vi "stave HDI measure shih v0.vi"() -> ()   [LabVIEW 2016]
uses:
  <vilib>/Utility/file.llb/Read Delimited Spreadsheet (DBL).vi
  <vilib>/Utility/file.llb/Write Delimited Spreadsheet (DBL).vi
  Classes/Controllers/Motion/Copy of Motion Folder/Motion.lvclass
  Classes/Controllers/Camera/Copy of Controller Folder/Controller.lvclass
panel:
  out "txt check":dbl[][](array[numeric])
  in  "north first switch":bool
  out "position from OGP all":dbl[][][](array[numeric]) format="%#_8g"
  out "HDI-stave deviation all":dbl[][][](array[numeric]) format="%#_8g"
  out "HDI - stave deviation on time":dbl[][](array[numeric]) format="%#_8g"
  out "position from OGP on time":dbl[][](array[numeric]) format="%#_8g"
  in  "default south HDI upper left":dbl[](array[numeric])=[448.322, 976.582, 74.9872, 0.000191129]
  in  "test":bool
  in  "how much HDI":i32=2
  out "bottom right":dbl[][](array[numeric]) format="%#_8g"
  out "bottom left":dbl[][](array[numeric]) format="%#_8g"
  out "top left":dbl[][](array[numeric]) format="%#_8g"
  out "HDI center position":dbl[][](array[numeric]) format="%#_8g"
  in  "default north HDI upper left":dbl[](array[numeric])=[448.322, 976.582, 74.9872, 0.000191129]
  in  "Default HDI size":dbl[](array[numeric])=[24.2437, 231.446, -0.099339, 0.000191129]
  out "measure times":dbl
  in  "Parking position":dbl[](array[numeric])=[625.0, 625.0, 0.0, 0.01]
  in  "measure HDI position":bool
  in  "calculate":bool
  in  "go to park":bool
  in  "stop":bool
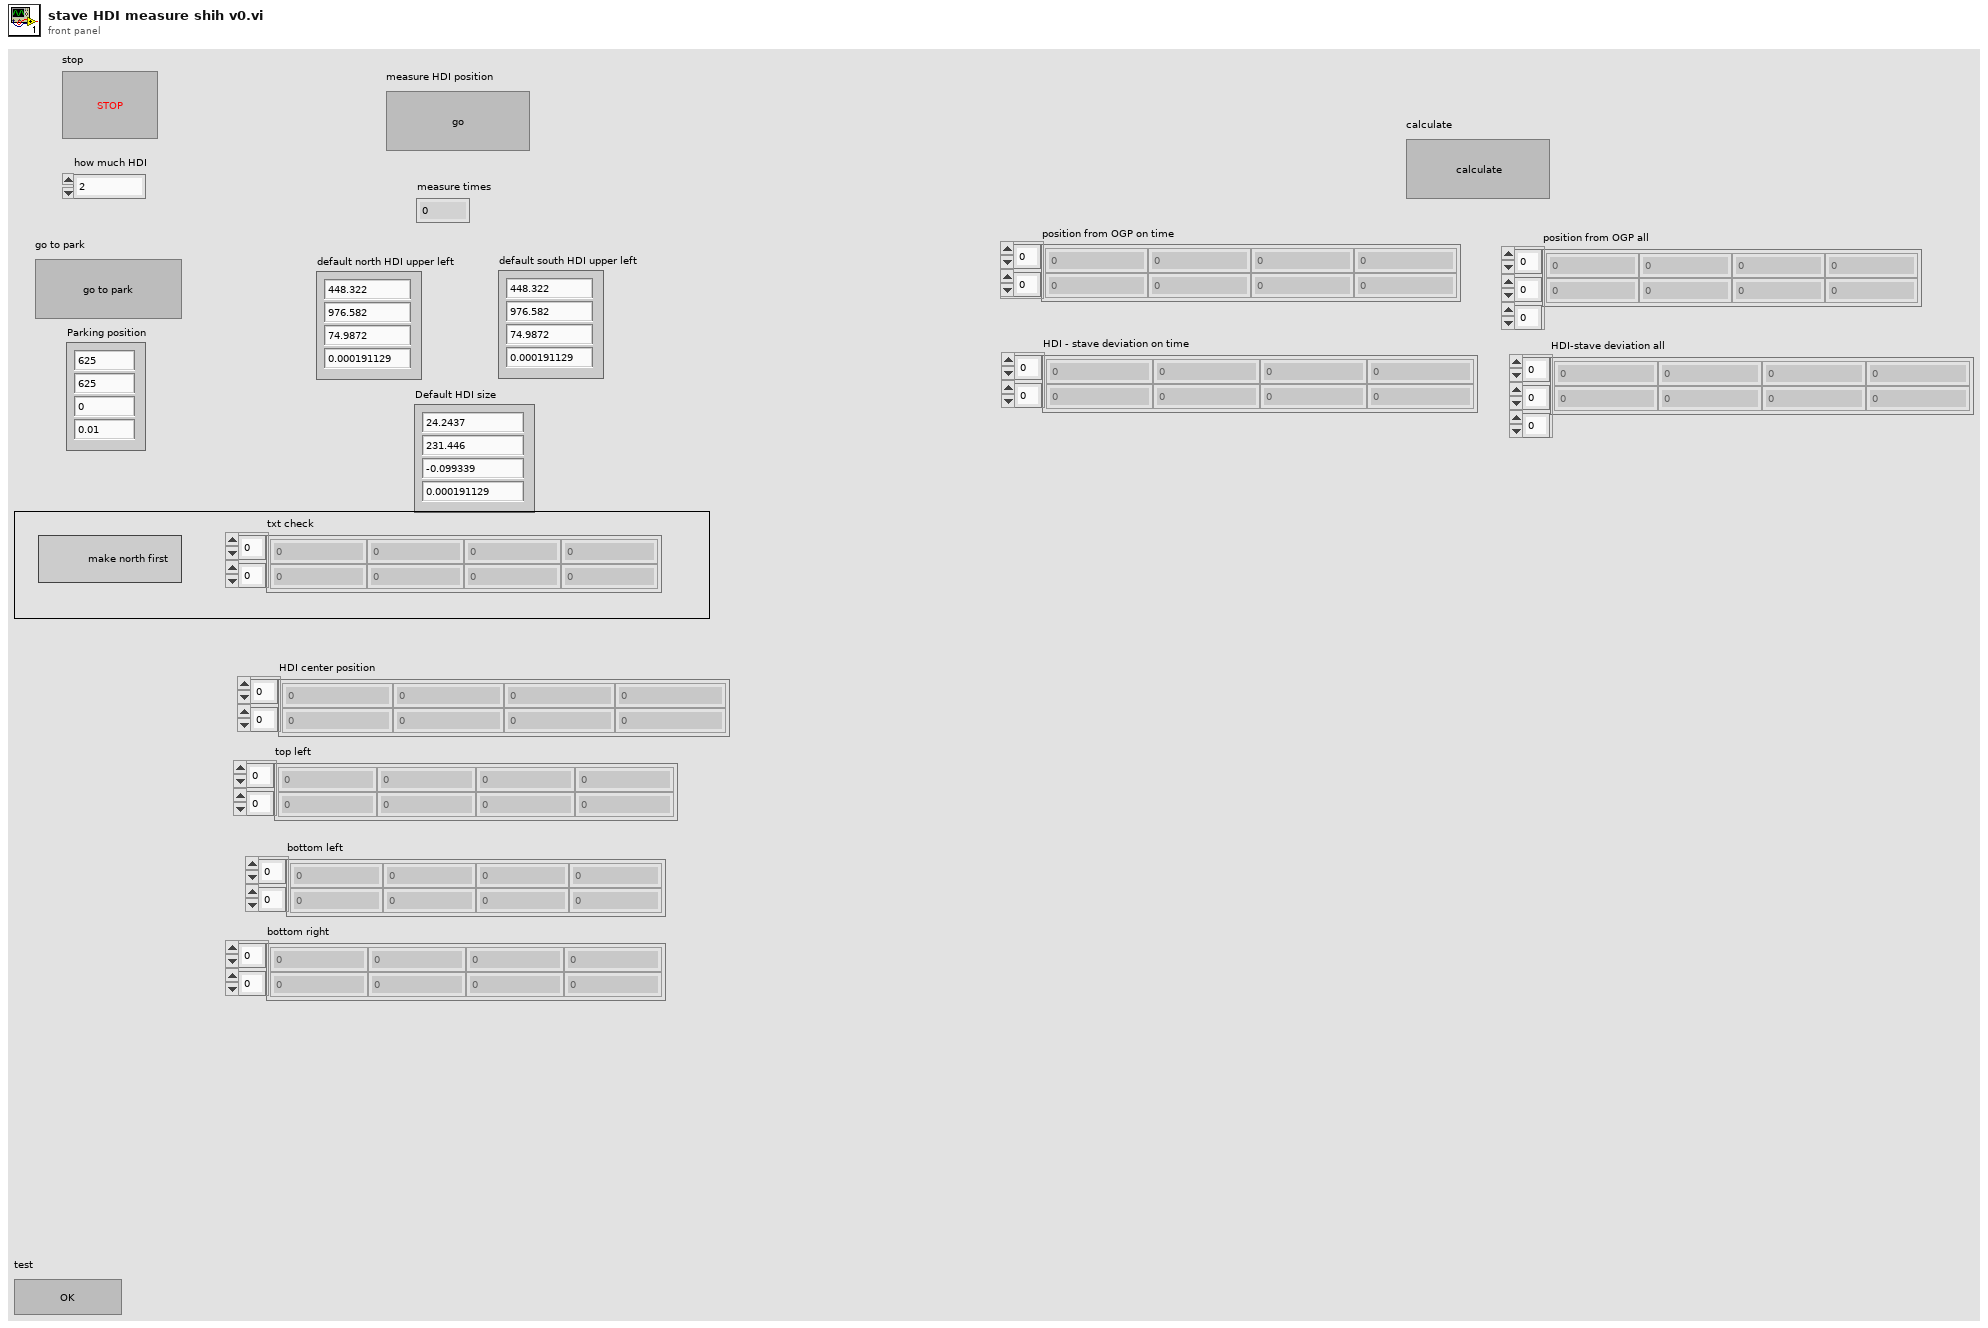
[diagram p1: front panel]
types:
  T1 = typedef "Controller.lvclass/Controllers.ctl" = cluster{"Copy of Motion.lvclass":refnum<class "Motion.lvclass">, "Copy of I-O.lvclass":refnum<class "I-O.lvclass">, "Copy of Dispenser.lvclass":refnum<class "Dispenser.lvclass">}
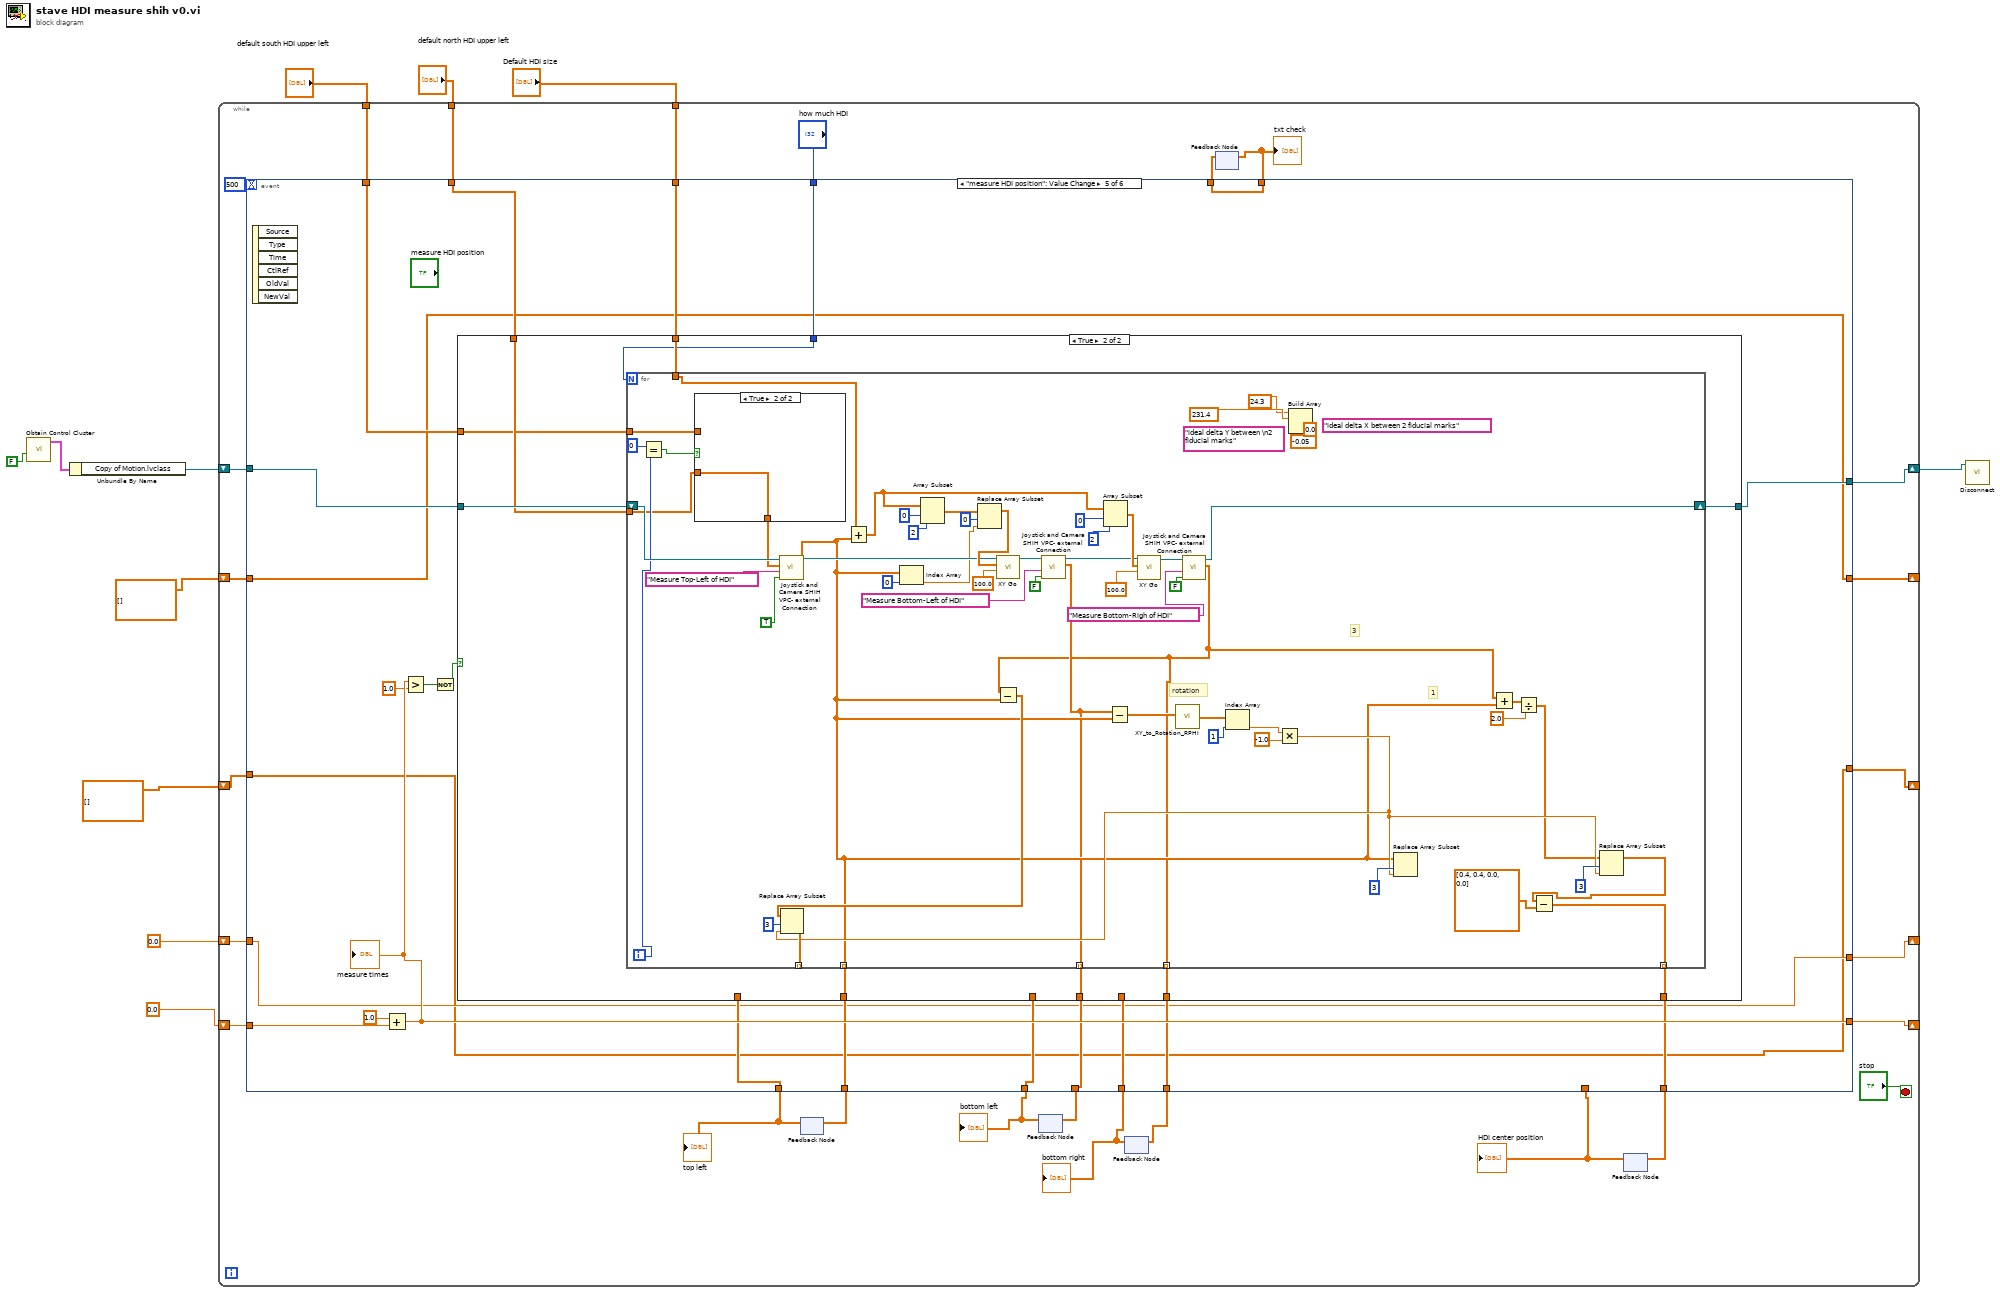
[diagram p0: block diagram]
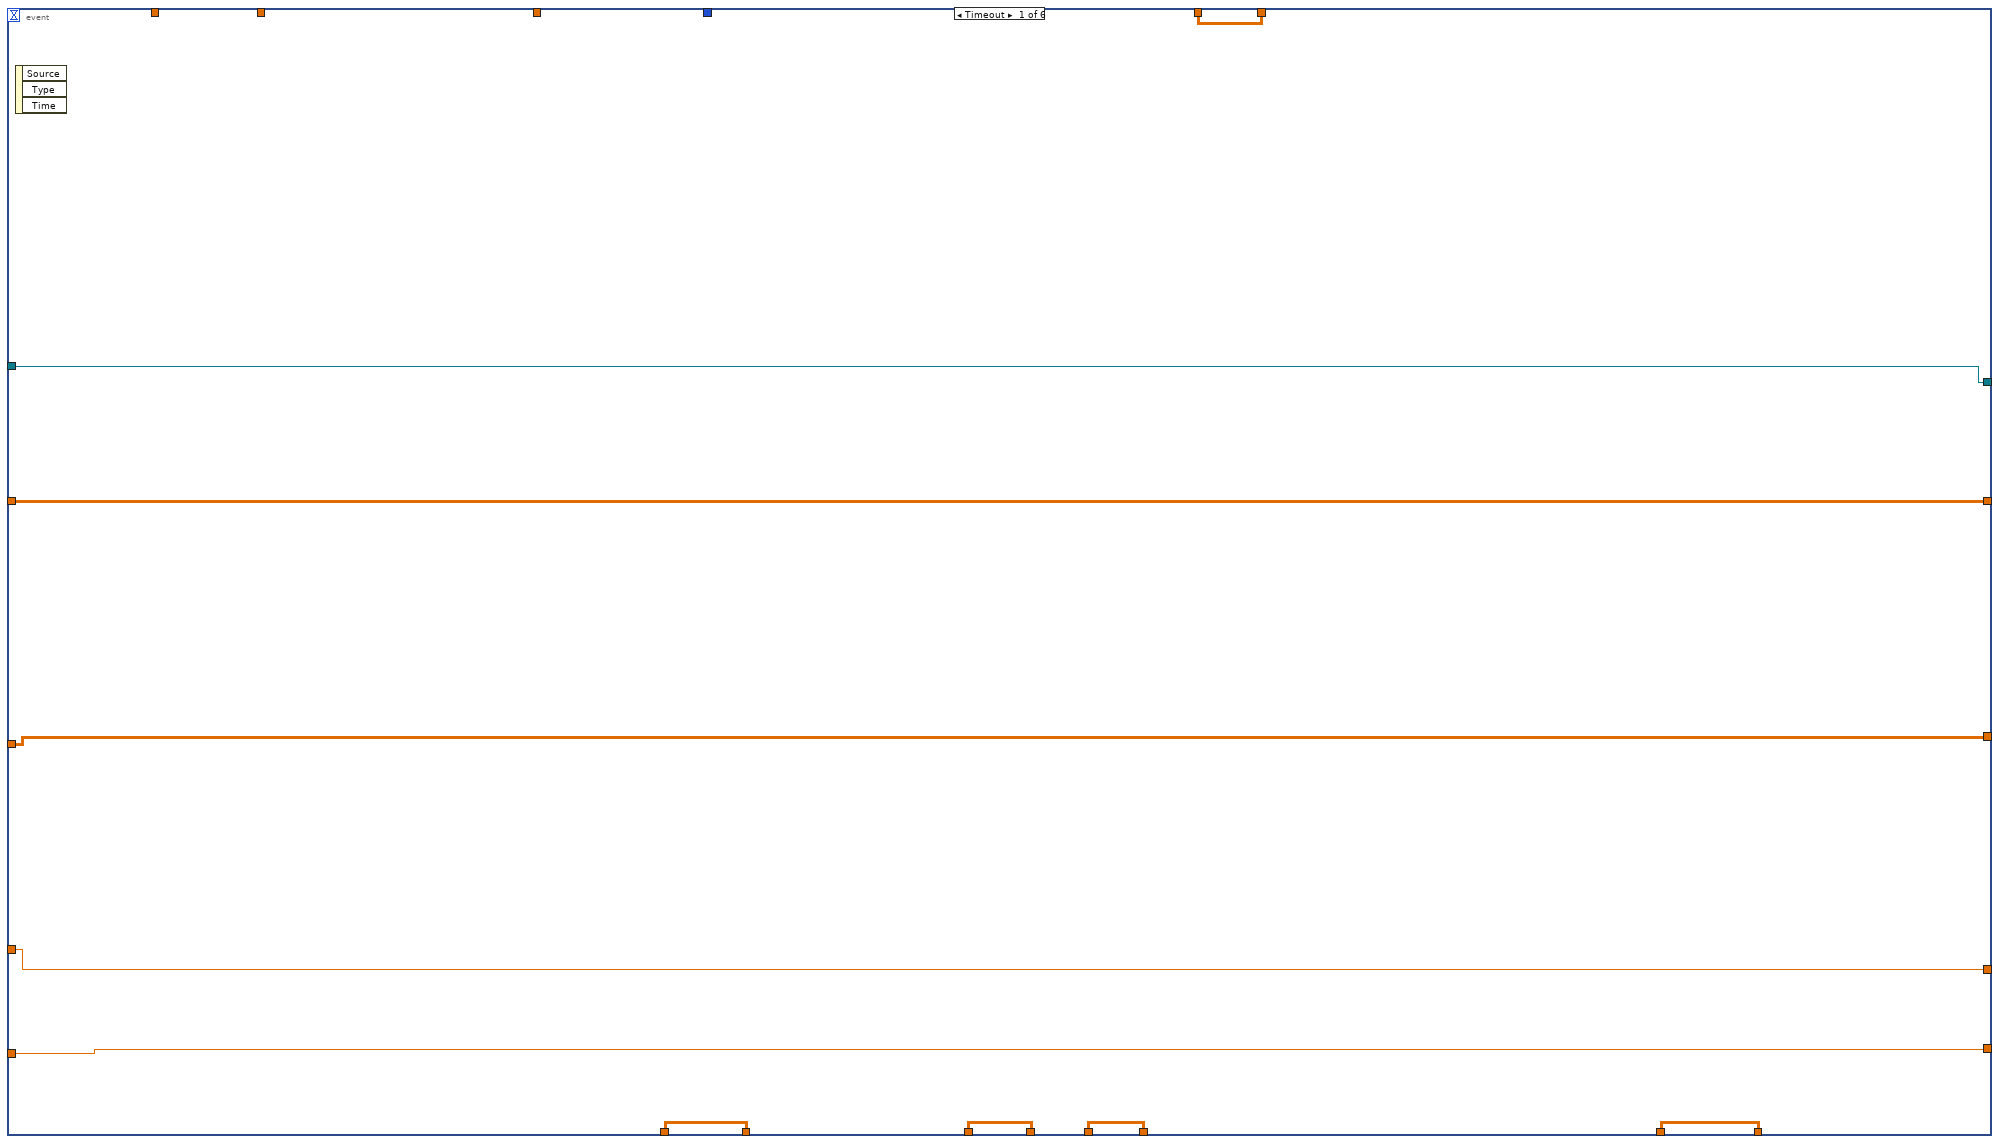
[diagram p2: hidden frame]
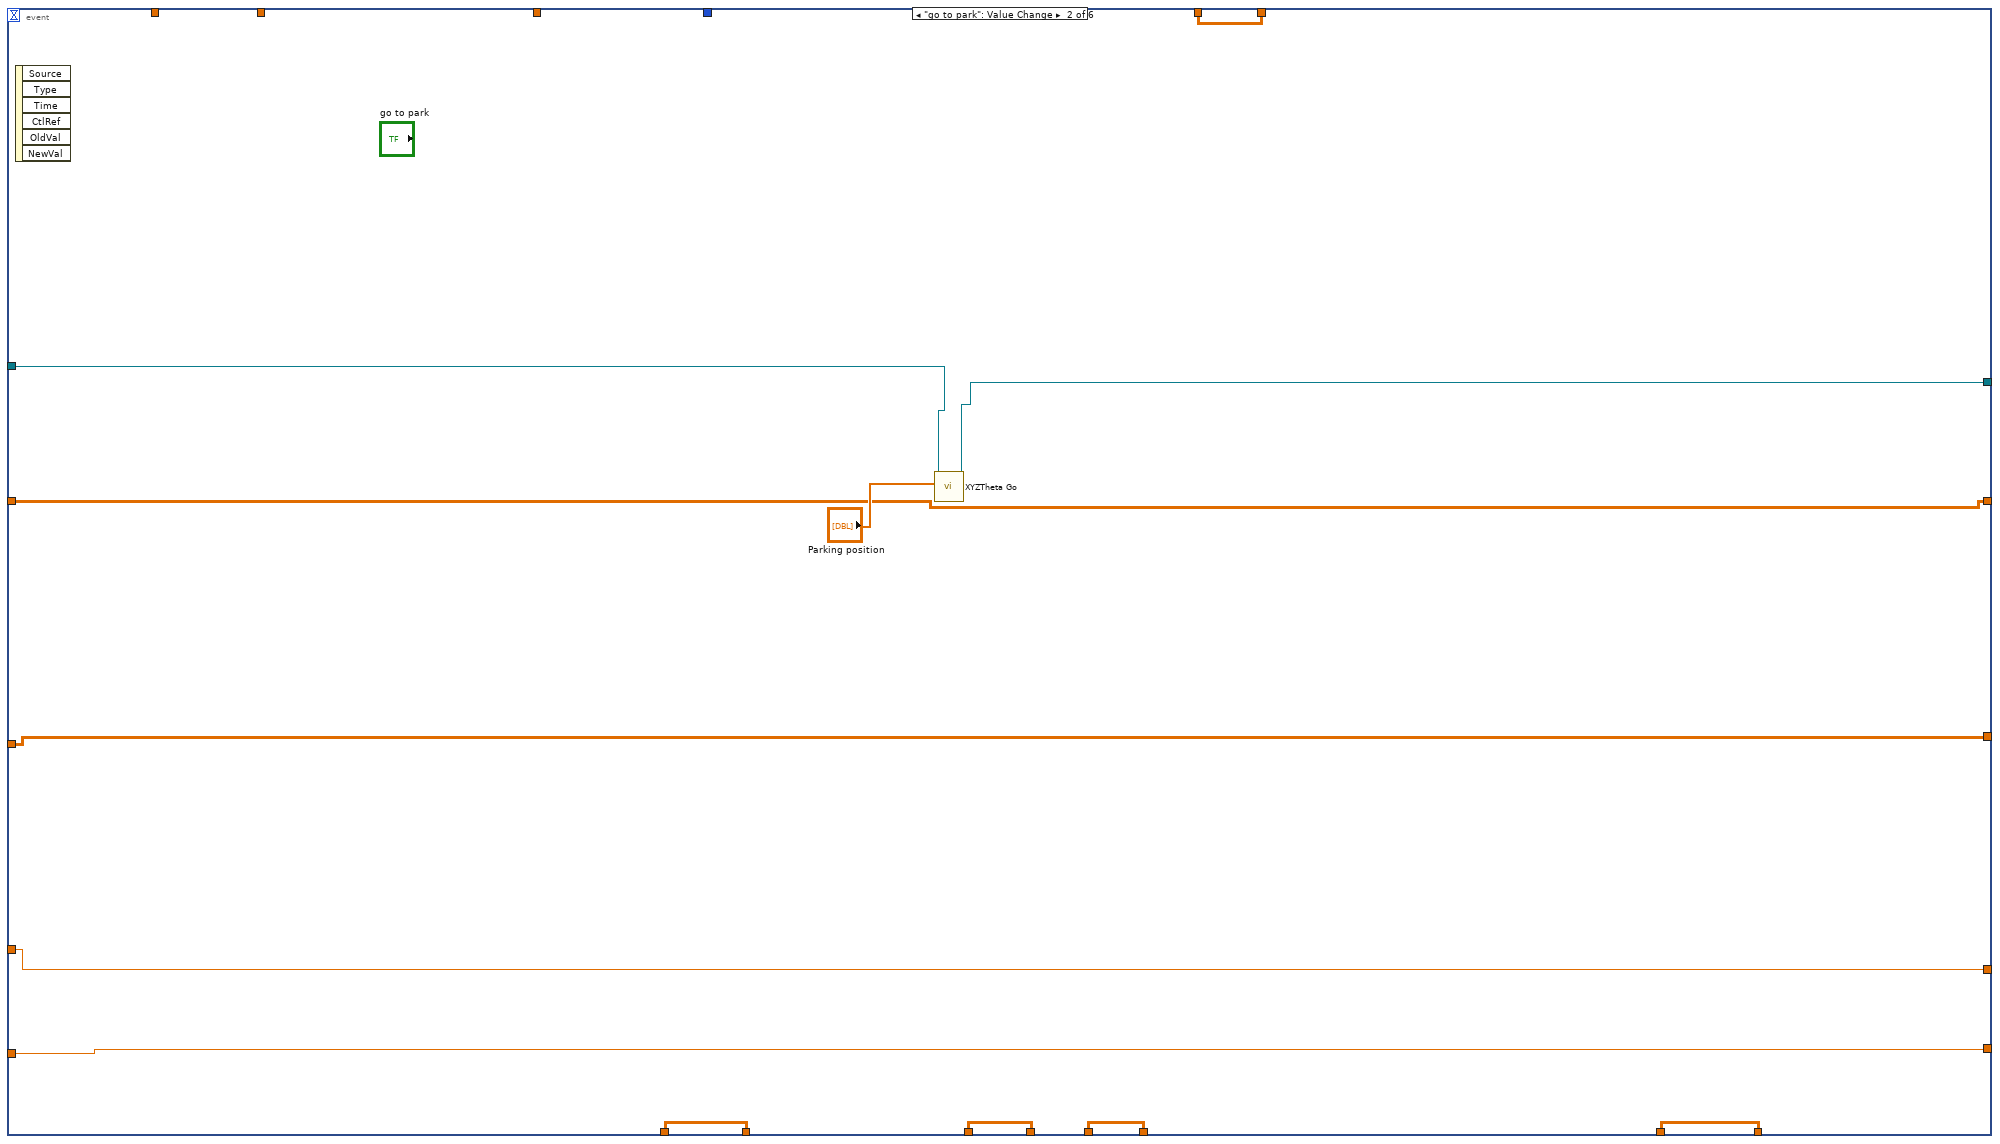
[diagram p3: hidden frame]
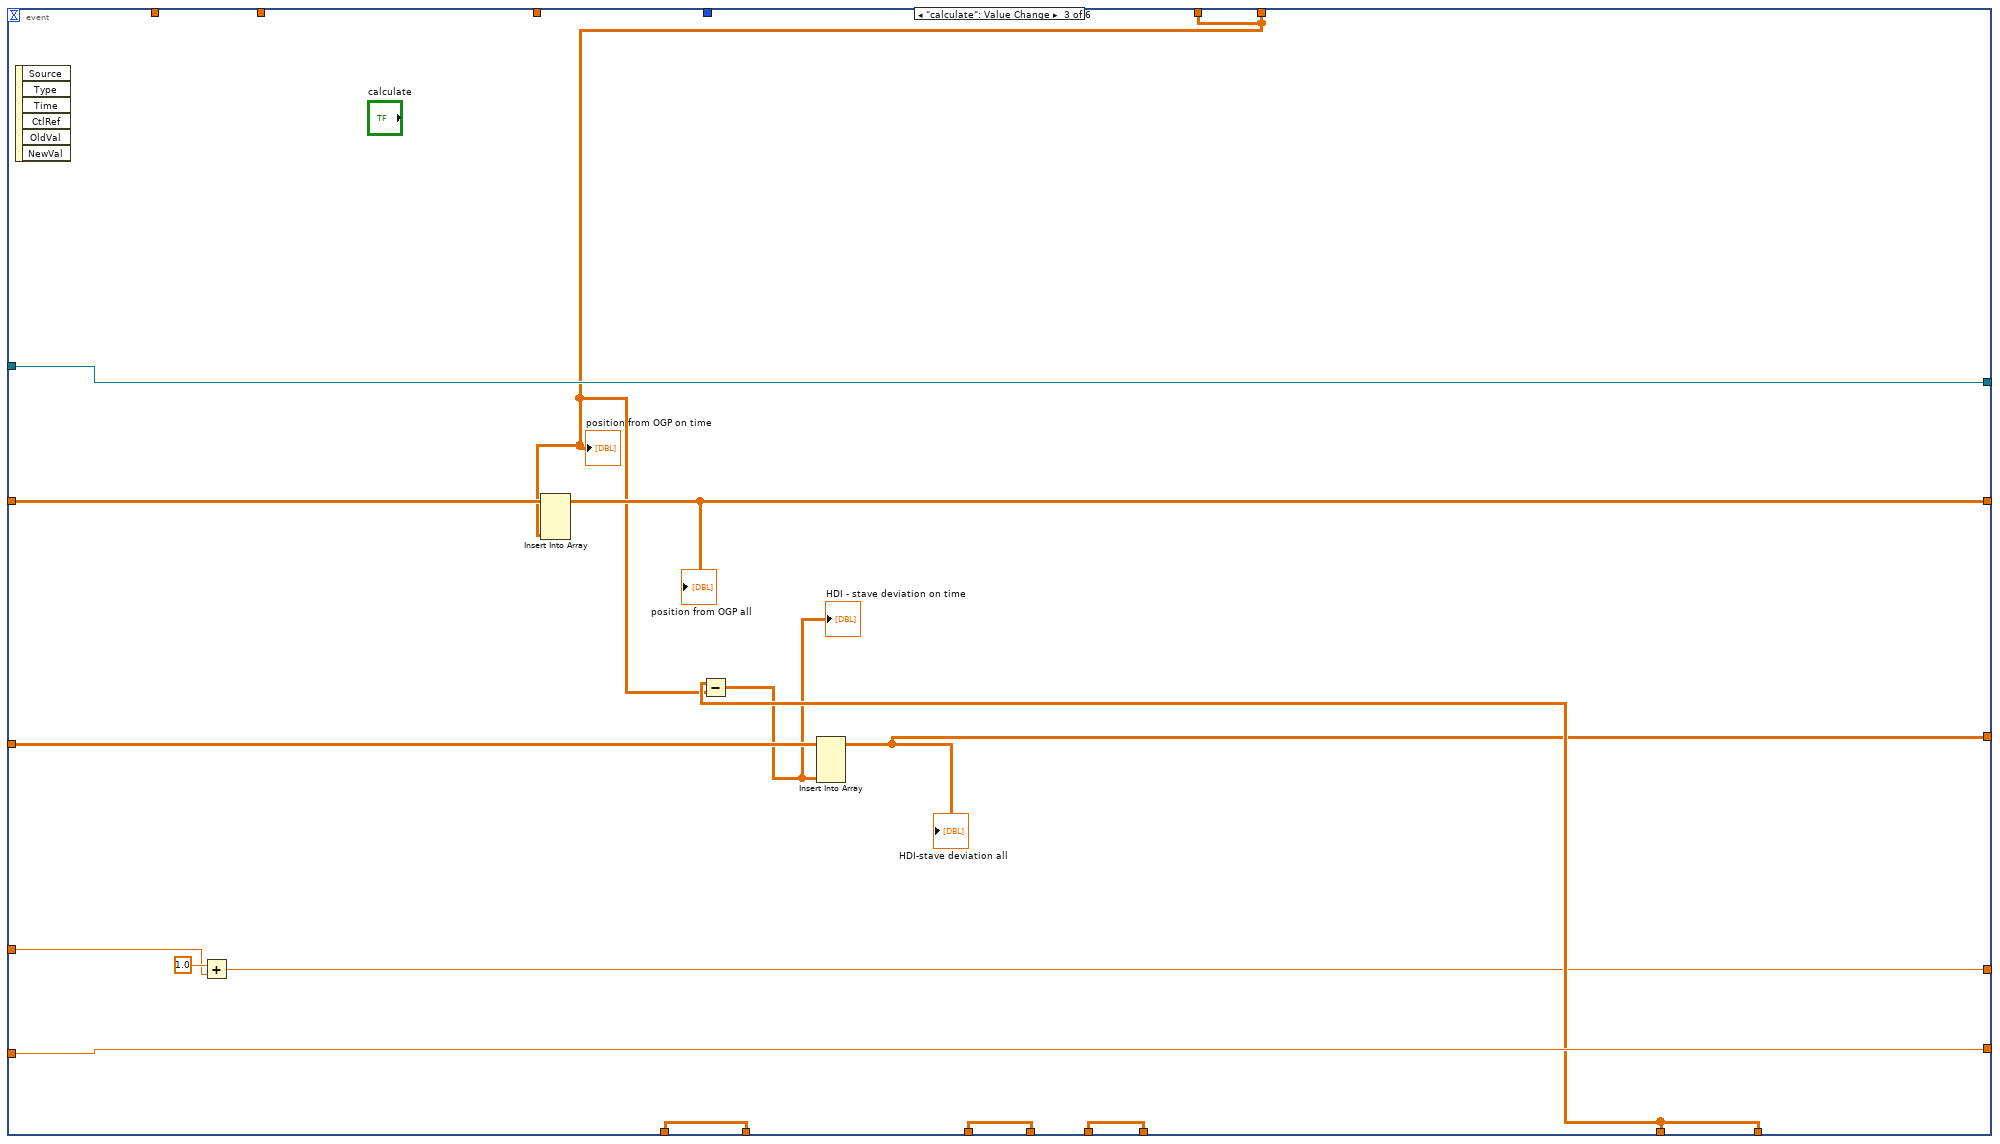
[diagram p4: hidden frame]
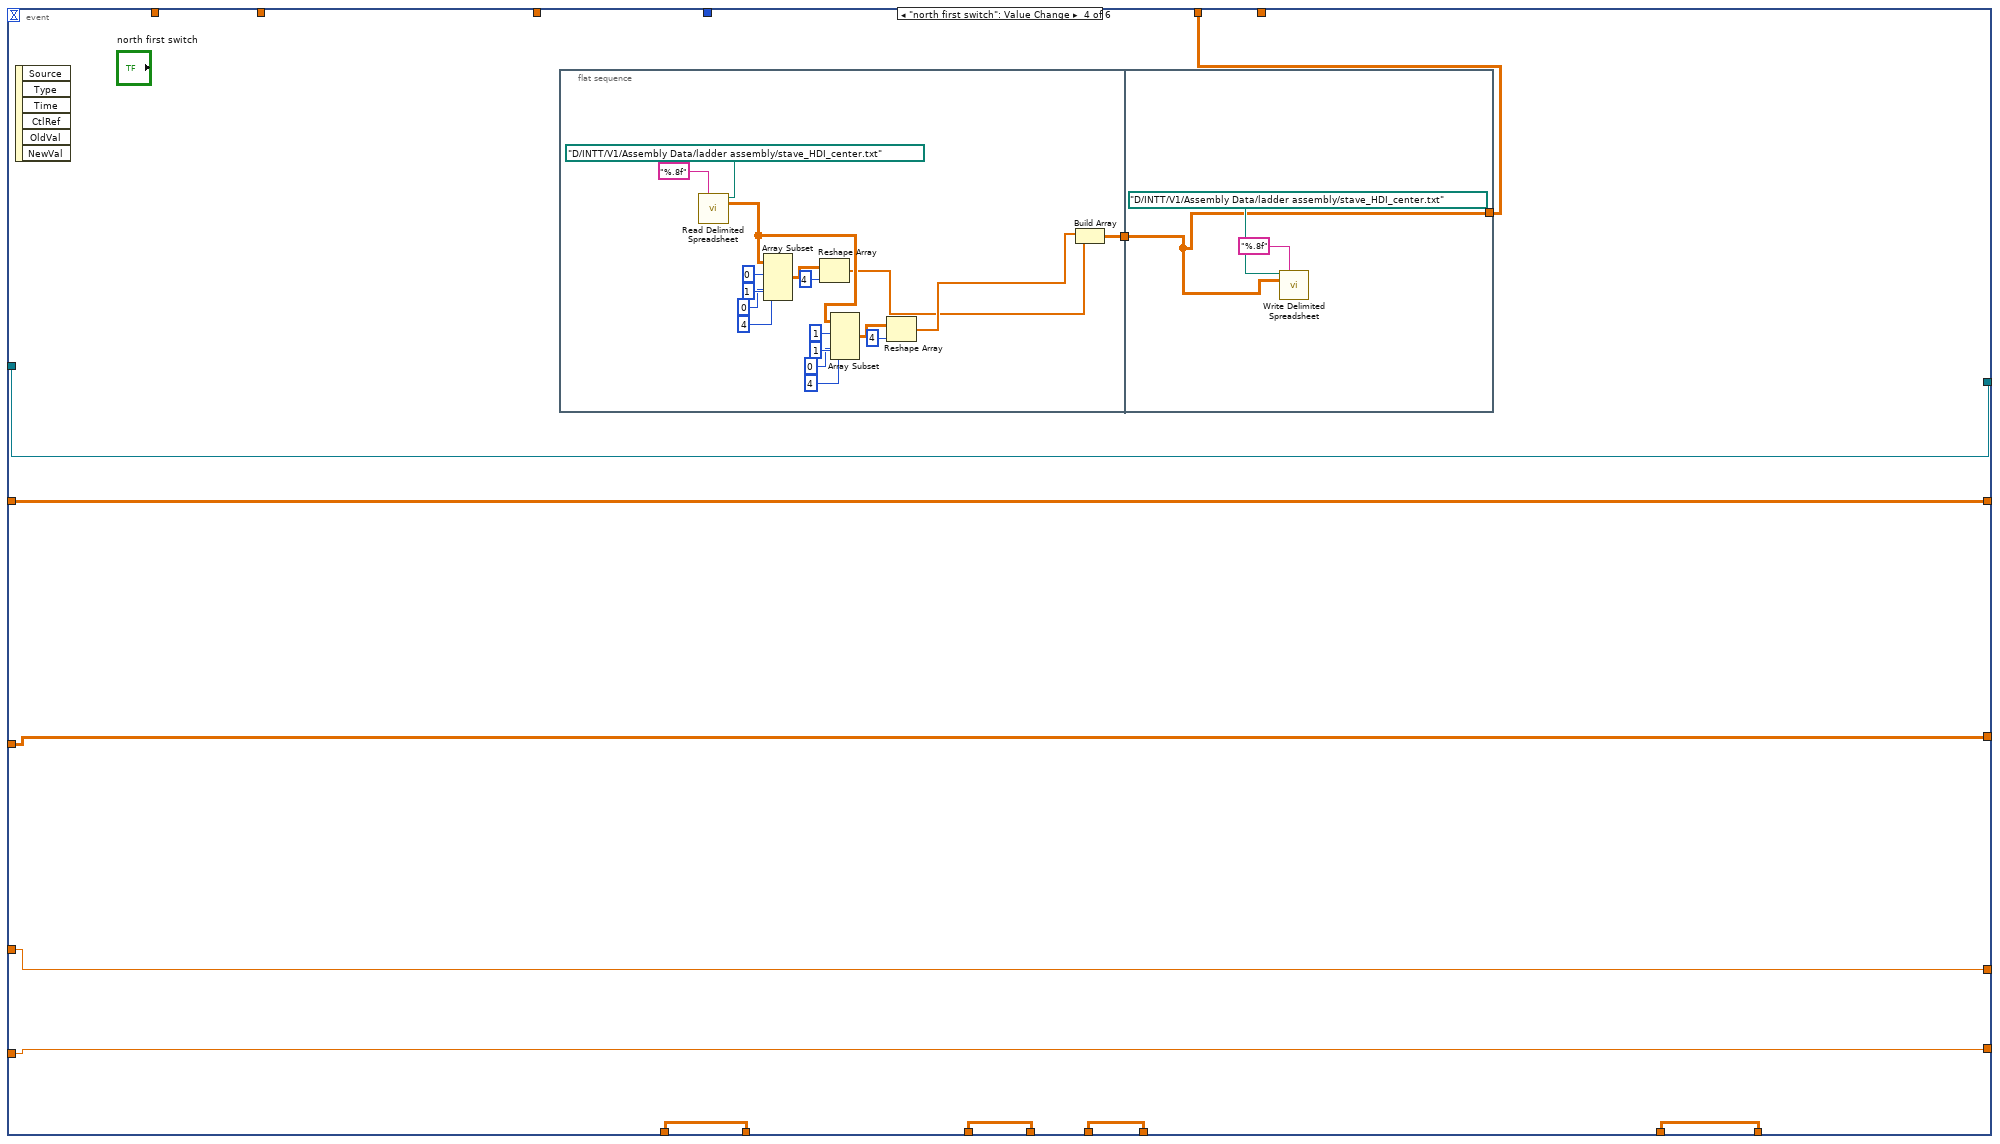
[diagram p5: hidden frame]
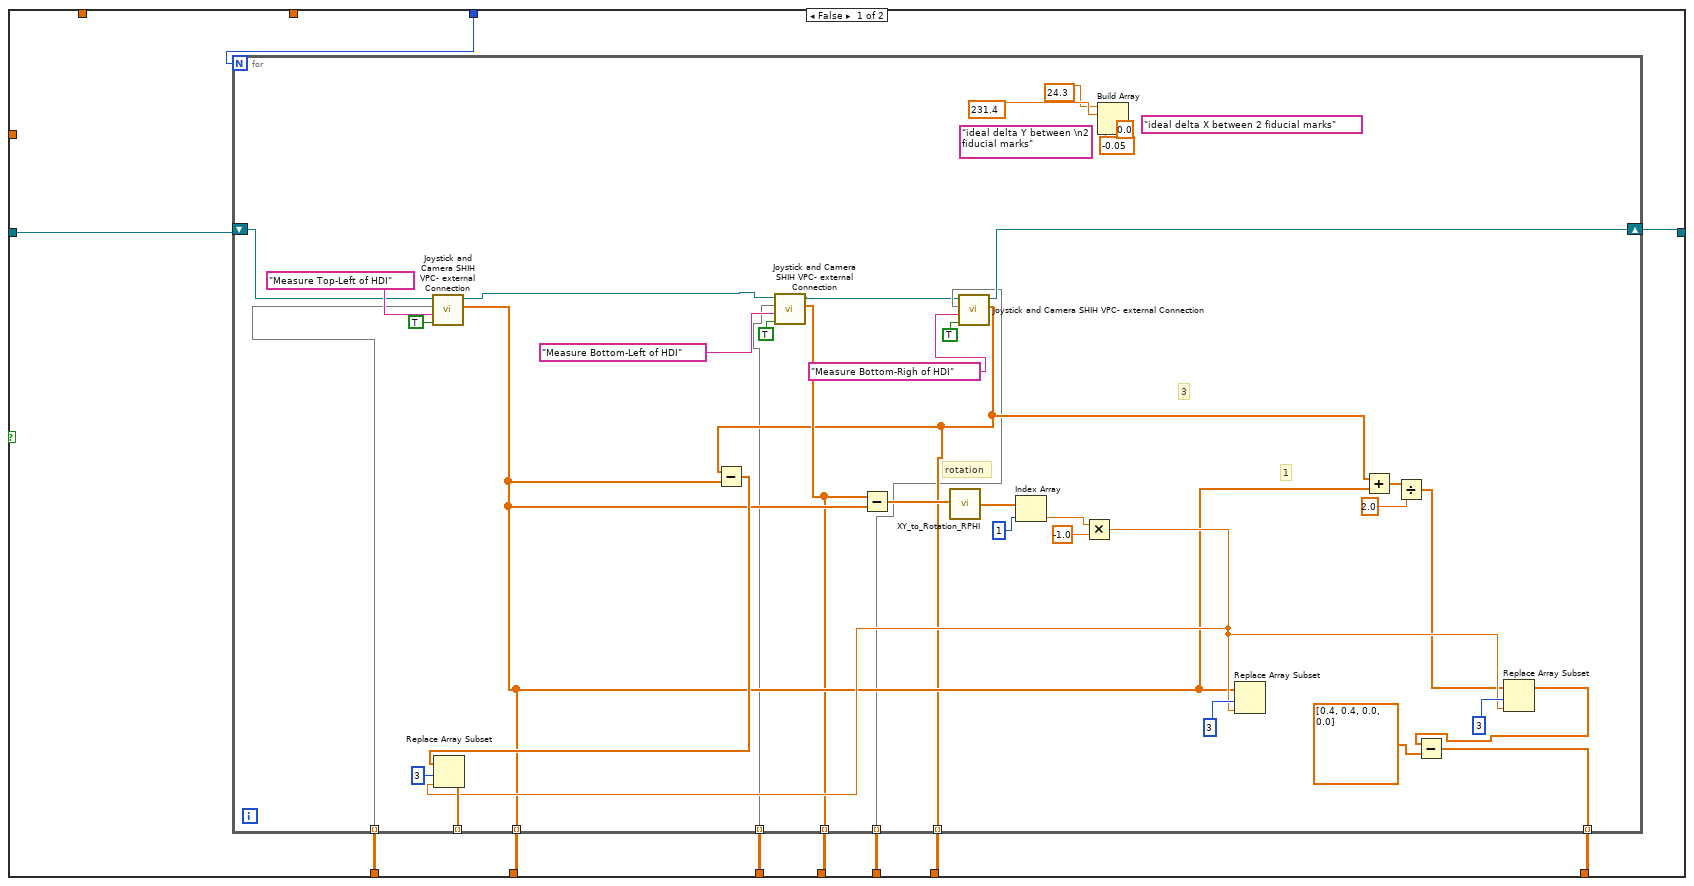
[diagram p6: hidden frame]
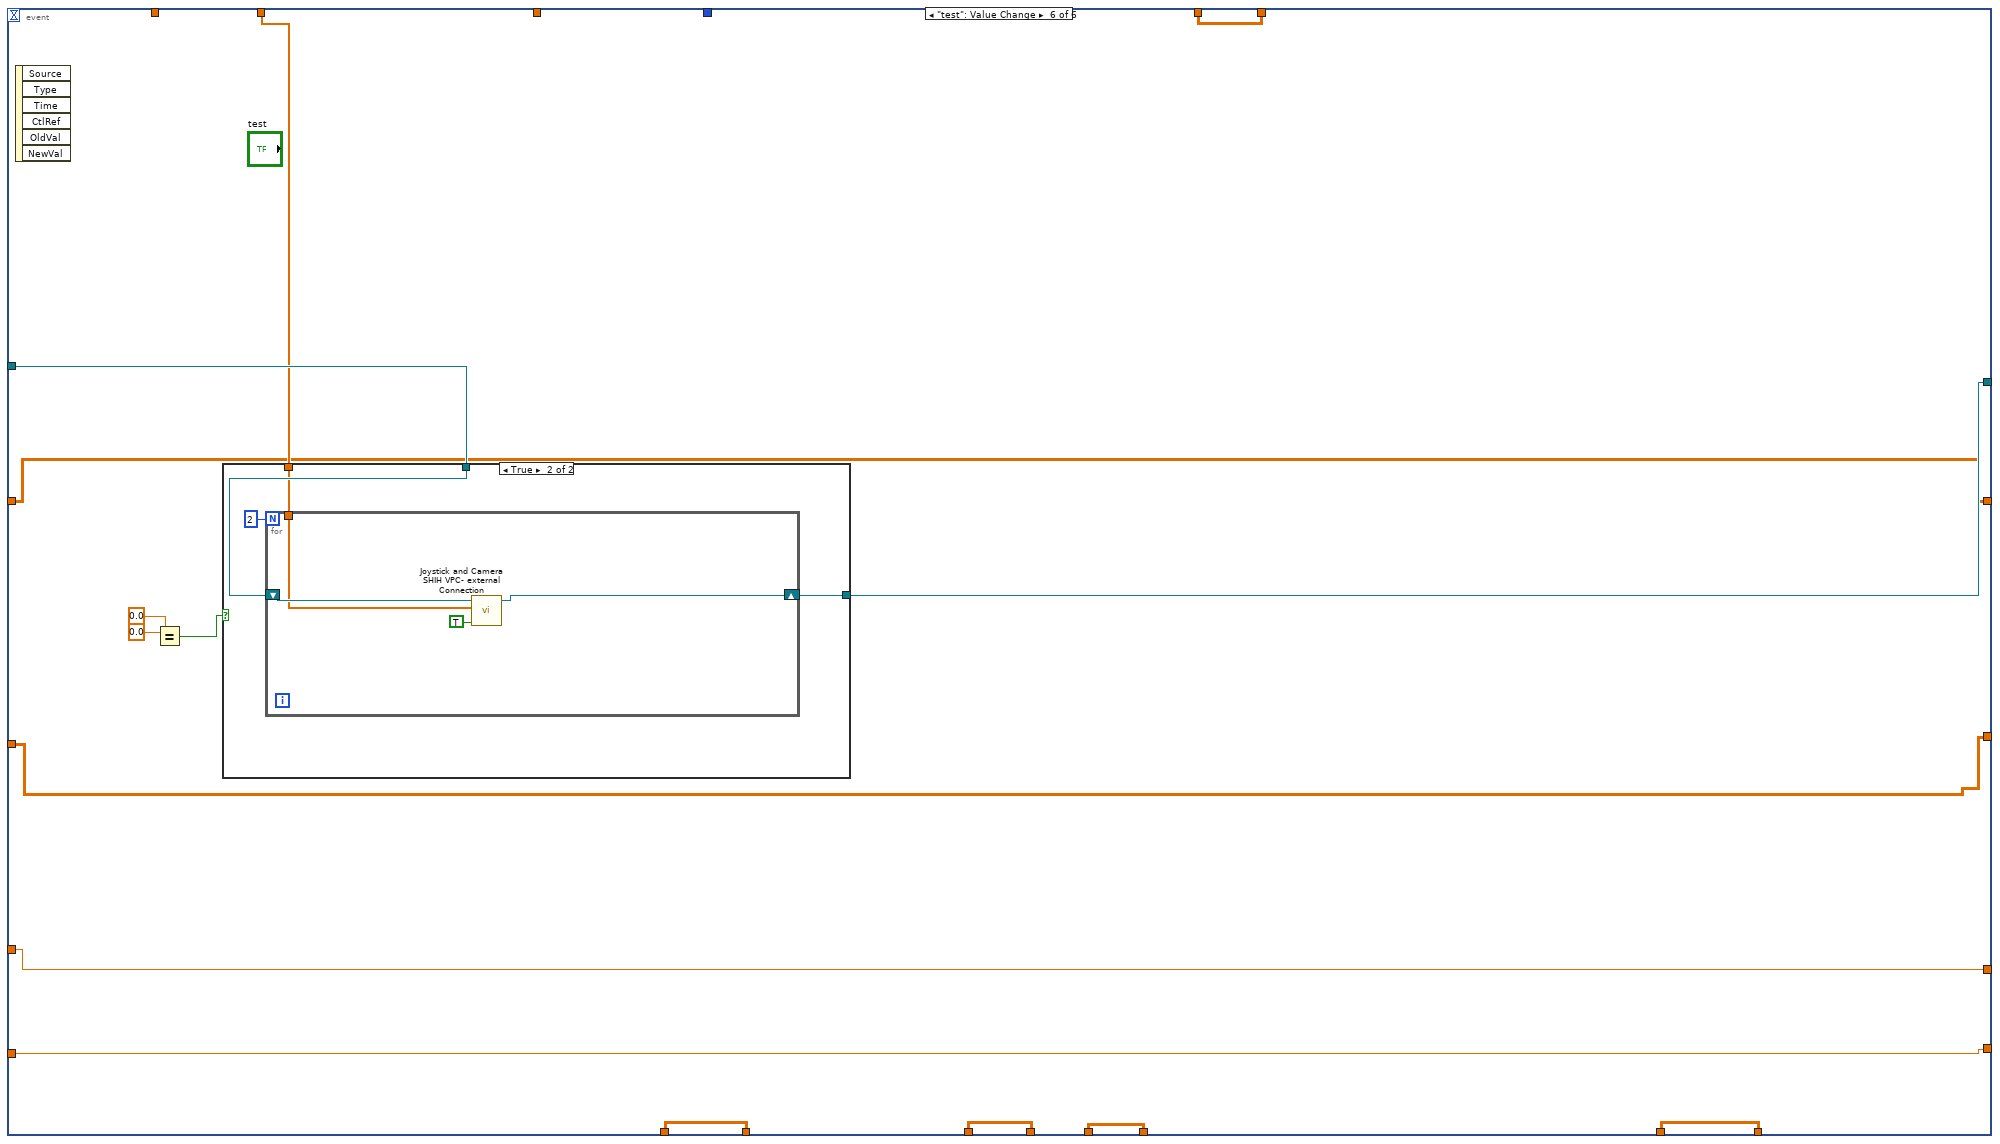
[diagram p8: hidden frame]
diagram:
  n1 = call "Obtain Control Cluster.vi"("I/O"=FALSE) -> ("Control Out"=w11:T1)  [unwired: 10 in]
  n2 = Unbundle By Name(w11) -> ("Copy of Motion.lvclass"=w9:refnum<class "Motion.lvclass">)
  n3 = while {
    shift-right: [w34] -> w8
    shift-left: w9 -> [w35]
    shift-right: [w32] -> _
    shift-left: 0.0 -> [w33]
    tunnel: "Default HDI size" -> [w31]
    tunnel: "default north HDI upper left" -> [w30]
    tunnel: "default south HDI upper left" -> [w21]
    shift-right: [w18] -> _
    shift-left: 0.0 -> [w19]
    shift-right: [w16] -> _
    shift-left: dbl[][][] [] -> [w17]
    shift-right: [w14] -> _
    shift-left: dbl[][][] [] -> [w15]
    stop <- "stop" stop-if-true
    n4 = feedback #1() -> (w27:dbl[][])  [unwired: 1 in]
    "top left" <- w27
    n5 = feedback #2() -> (w24:dbl[][])  [unwired: 1 in]
    "bottom left" <- w24
    n6 = feedback #3() -> (w23:dbl[][])  [unwired: 1 in]
    "bottom right" <- w23
    n7 = feedback #4() -> (w12:dbl[][])  [unwired: 1 in]
    "txt check" <- w12
    n8 = feedback #5() -> (w20:dbl[][])  [unwired: 1 in]
    "HDI center position" <- w20
    n9 = event shown="[4] \"measure HDI position\": Value Change" {
      selector: _ -> [_ _ _ _ _ _]
      dyn-events: _ -> [_ _ _ _ _ _]
      timeout: 500 -> [_ _ _ _ _ _]
      tunnel: w35 -> [w47 w58 w74 w85 w129 w259]
      tunnel: [w47 w57 w74 w85 w113 w258] -> w34
      tunnel: w33 -> [w42 w52 w70 w81 w128 w257]
      tunnel: [w42 w52 w70 w81 w126 w257] -> w32
      tunnel: w31 -> [_ _ _ _ w122 _]
      tunnel: w30 -> [_ _ _ _ w121 w256]
      tunnel: [w46 w56 w69 w77 w120 w249] -> w29
      tunnel: w20 -> [w46 w56 w69 w77 _ w249]
      tunnel: [w45 w55 w73 w80 w119 w252] -> w28
      tunnel: w27 -> [w45 w55 w73 w80 w116 w252]
      tunnel: [w44 w54 w72 w79 w118 w251] -> w26
      tunnel: [w43 w53 w71 w78 w117 w250] -> w25
      tunnel: w24 -> [w44 w54 w72 w79 w115 w251]
      tunnel: w23 -> [w43 w53 w71 w78 w114 w250]
      tunnel: "how much HDI" -> [_ _ _ _ w112 _]
      tunnel: w21 -> [_ _ _ _ w111 _]
      tunnel: w19 -> [w41 w51 w67 w82 w110 w248]
      tunnel: [w41 w51 w66 w82 w110 w248] -> w18
      tunnel: w17 -> [w39 w49 w65 w83 w108 w247]
      tunnel: [w39 w49 w64 w83 w108 w247] -> w16
      tunnel: w15 -> [w40 w50 w63 w84 w109 w246]
      tunnel: [w40 w50 w62 w84 w109 w246] -> w14
      tunnel: [w38 w48 w60 w75 w107 w245] -> w13
      tunnel: w12 -> [w38 w48 w60 _ w107 w245]
      event Timeout {
        n10 = event-data() -> ()  [unwired: 1 in, 3 out]
      }
      event "go to park": Value Change {
        n11 = event-data() -> ()  [unwired: 1 in, 6 out]
        n12 = call "XYZTheta Go.vi"("XYZTheta In"="Parking position", "Motion in"=w58) -> ("Motion out"=w57:refnum<class "Motion.lvclass">)  [unwired: 7 in, 2 out]
      }
      event "calculate": Value Change {
        n13 = event-data() -> ()  [unwired: 1 in, 6 out]
        n14 = Add(x=1.0, y=w67) -> (x+y=w66:dbl)
        n15 = Insert Into Array(array=w63, new element=w60) -> (w62:dbl[][][])  [unwired: 3 in]
        "position from OGP all" <- w62
        n16 = Subtract(x=w69, y=w60) -> (x-y=w61:dbl[][])
        "HDI - stave deviation on time" <- w61
        n17 = Insert Into Array(array=w65, new element=w61) -> (w64:dbl[][][])  [unwired: 3 in]
        "HDI-stave deviation all" <- w64
        "position from OGP on time" <- w60
      }
      event "north first switch": Value Change {
        n18 = event-data() -> ()  [unwired: 1 in, 6 out]
        n19 = flat-sequence {
          tunnel: [w89] -> w76
          tunnel: w76 -> [w104]
          tunnel: [w104] -> w75
          frame #0 {
            n20 = call-poly <vilib>:"Read Delimited Spreadsheet.vi"("file path (dialog if empty)"=path "D:/INTT/V1/Assembly Data/ladder assembly/stave_HDI_center.txt" ("file path (dialog if empty) 3"), "format (%.3f)"="%.8f") -> ("all rows"=w90:dbl[][])  [unwired: 8 in, 5 out]
            n21 = Array Subset(array=w90, index (row)=0 ("index"), length (row)=1 ("length"), index (col)=0 ("index"), length (col)=4 ("length")) -> (w100:dbl[][])
            n22 = Reshape Array(w100, 4 ("dimension size")) -> (w87:dbl[])
            n23 = Array Subset(array=w90, index (row)=1 ("index"), length (row)=1 ("length"), index (col)=0 ("index"), length (col)=4 ("length")) -> (w94:dbl[][])
            n24 = Reshape Array(w94, 4 ("dimension size")) -> (w88:dbl[])
            n25 = Build Array(w88, w87) -> (w89:dbl[][])
          }
          frame #1 {
            n26 = call-poly <vilib>:"Write Delimited Spreadsheet.vi"("file path (dialog if empty)"=path "D:/INTT/V1/Assembly Data/ladder assembly/stave_HDI_center.txt" ("file path (dialog if empty) 4"), "format (%.3f)"="%.8f", "2D data"=w104) -> ()  [unwired: 11 in, 2 out]
          }
        }
      }
      event "measure HDI position": Value Change {
        n27 = event-data() -> ()  [unwired: 1 in, 6 out]
        n28 = Add(x=1.0, y=w128) -> (x+y=w126:dbl)
        "measure times" <- w126
        n29 = Greater?(x=w126, y=1.0) -> (0:w124:bool)
        n30 = Not(x=w124) -> (.not. x?=w123:bool)
        n31 = case shown="True" w123 {
          tunnel: w129 -> [w131 w186]
          tunnel: [w132 w179] -> w113
          tunnel: w122 -> [_ w185]
          tunnel: w121 -> [_ w184]
          tunnel: [w136 w183] -> w120
          tunnel: [w139 w182] -> w119
          tunnel: [w138 w181] -> w118
          tunnel: [w137 w180] -> w117
          tunnel: w116 -> [w135 _]
          tunnel: w115 -> [w134 _]
          tunnel: w114 -> [w133 _]
          tunnel: w112 -> [w130 w178]
          tunnel: w111 -> [_ w177]
          frame False {
            n32 = for {
              N: w130 -> [_]
              shift-right: [w157] -> w132
              shift-left: w131 -> [w158]
              tunnel: [w173] -> _ mode=indexing
              tunnel: [w149] -> w136 mode=indexing
              tunnel: [w148] -> w139 mode=indexing
              tunnel: [w147] -> w138 mode=indexing
              tunnel: [w146] -> w137 mode=indexing
              tunnel: w135 -> [w144] mode=indexing
              tunnel: w134 -> [w142] mode=indexing
              tunnel: w133 -> [w141] mode=indexing
              (unwired) "ideal delta Y between \n2 fiducial marks"
              (unwired) "ideal delta X between 2 fiducial marks"
              # "rotation"
              # "1"
              # "3"
              n33 = call "Joystick and Camera SHIH VPC- external Connection.vi"("Motion in"=w158, "XYZTheta"=w144, "Measurement Point"="Measure Top-Left of HDI", "Inital GO"=TRUE) -> ("Motion out"=w143:refnum<class "Motion.lvclass">, "Sum"=w148:dbl[])  [unwired: 3 in, 2 out]
              n34 = call "Joystick and Camera SHIH VPC- external Connection.vi"("Motion in"=w143, "XYZTheta"=w142, "Measurement Point"="Measure Bottom-Left of HDI", "Inital GO"=TRUE) -> ("Motion out"=w140:refnum<class "Motion.lvclass">, "Sum"=w147:dbl[])  [unwired: 3 in, 2 out]
              n35 = Subtract(x=w147, y=w148) -> (x-y=w166:dbl[])
              n36 = call "XY_to_Rotation_RPHI.vi"("X-Y"=w166) -> ("r-phi"=w162:dbl[])
              n37 = call "Joystick and Camera SHIH VPC- external Connection.vi"("Motion in"=w140, "XYZTheta"=w141, "Measurement Point"="Measure Bottom-Righ of HDI", "Inital GO"=TRUE) -> ("Motion out"=w157:refnum<class "Motion.lvclass">, "Sum"=w146:dbl[])  [unwired: 3 in, 2 out]
              n38 = Subtract(x=w146, y=w148) -> (x-y=w155:dbl[])
              n39 = Index Array(array=w162, index=1) -> (element=w159:dbl)
              n40 = Multiply(x=w159, y=-1.0) -> (x*y=w153:dbl)
              n41 = Replace Array Subset(array=w155, new element=w153, index=3) -> (w173:dbl[])
              n42 = Build Array(24.3 ("y"), 231.4 ("y"), 0.0 ("element"), -0.05 ("element")) -> ()  [unwired: 1 out]
              n43 = Replace Array Subset(array=w148, new element=w153, index=3) -> ()  [unwired: 1 out]
              n44 = Add(x=w146, y=w148) -> (x+y=w175:dbl[])
              n45 = Divide(x=w175, y=2.0) -> (x/y=w152:dbl[])
              n46 = Replace Array Subset(array=w152, new element=w153, index=3) -> (w150:dbl[])
              n47 = Subtract(x=w150, y=dbl[] [0.4, 0.4, 0.0, 0.0]) -> (x-y=w149:dbl[])
            }
          }
          frame True {
            n48 = for {
              N: w178 -> [_]
              tunnel: w185 -> [w207]
              shift-right: [w205] -> w179
              shift-left: w186 -> [w206]
              tunnel: w184 -> [w189]
              tunnel: [w239] -> _ mode=indexing
              tunnel: [w197] -> w183 mode=indexing
              tunnel: [w196] -> w182 mode=indexing
              tunnel: [w195] -> w181 mode=indexing
              tunnel: [w194] -> w180 mode=indexing
              tunnel: w177 -> [w187]
              i -> [w191]
              (unwired) "ideal delta Y between \n2 fiducial marks"
              (unwired) "ideal delta X between 2 fiducial marks"
              # "rotation"
              # "1"
              # "3"
              n49 = Equal?(x=0, y=w191) -> (x = y?=w192:bool)
              n50 = case shown="True" w192 {
                tunnel: [w243 w244] -> w188
                tunnel: w189 -> [_ w244]
                tunnel: w187 -> [w243 _]
                frame False {
                }
                frame True {
                }
              }
              n51 = call "Joystick and Camera SHIH VPC- external Connection.vi"("Motion in"=w206, "XYZTheta"=w188, "Measurement Point"="Measure Top-Left of HDI", "Inital GO"=TRUE) -> ("Motion out"=w219:refnum<class "Motion.lvclass">, "Sum"=w196:dbl[])  [unwired: 3 in, 2 out]
              n52 = Add(x=w207, y=w196) -> (x+y=w223:dbl[])
              n53 = Index Array(array=w196, index=0) -> (element=w210:dbl)
              n54 = Array Subset(array=w223, index=0, length=2) -> (w222:dbl[])
              n55 = Replace Array Subset(array=w222, new element=w210, index=0) -> (w220:dbl[])
              n56 = call-dynamic "XY Go.vi"("Speed"=100.0, "XY"=w220, "Motion in"=w219) -> ("Motion out"=w227:refnum<class "Motion.lvclass">)  [unwired: 7 in, 1 out]
              n57 = call "Joystick and Camera SHIH VPC- external Connection.vi"("Motion in"=w227, "Measurement Point"="Measure Bottom-Left of HDI", "Inital GO"=FALSE) -> ("Motion out"=w218:refnum<class "Motion.lvclass">, "Sum"=w195:dbl[])  [unwired: 4 in, 2 out]
              n58 = Array Subset(array=w223, index=0, length=2) -> (w233:dbl[])
              n59 = Subtract(x=w195, y=w196) -> (x-y=w217:dbl[])
              n60 = call-dynamic "XY Go.vi"("Speed"=100.0, "XY"=w233, "Motion in"=w218) -> ("Motion out"=w237:refnum<class "Motion.lvclass">)  [unwired: 7 in, 1 out]
              n61 = call "XY_to_Rotation_RPHI.vi"("X-Y"=w217) -> ("r-phi"=w213:dbl[])
              n62 = call "Joystick and Camera SHIH VPC- external Connection.vi"("Motion in"=w237, "Measurement Point"="Measure Bottom-Righ of HDI", "Inital GO"=FALSE) -> ("Motion out"=w205:refnum<class "Motion.lvclass">, "Sum"=w194:dbl[])  [unwired: 4 in, 2 out]
              n63 = Subtract(x=w194, y=w196) -> (x-y=w203:dbl[])
              n64 = Index Array(array=w213, index=1) -> (element=w208:dbl)
              n65 = Multiply(x=w208, y=-1.0) -> (x*y=w201:dbl)
              n66 = Replace Array Subset(array=w203, new element=w201, index=3) -> (w239:dbl[])
              n67 = Build Array(24.3 ("y"), 231.4 ("y"), 0.0 ("element"), -0.05 ("element")) -> ()  [unwired: 1 out]
              n68 = Replace Array Subset(array=w196, new element=w201, index=3) -> ()  [unwired: 1 out]
              n69 = Add(x=w194, y=w196) -> (x+y=w241:dbl[])
              n70 = Divide(x=w241, y=2.0) -> (x/y=w200:dbl[])
              n71 = Replace Array Subset(array=w200, new element=w201, index=3) -> (w198:dbl[])
              n72 = Subtract(x=w198, y=dbl[] [0.4, 0.4, 0.0, 0.0]) -> (x-y=w197:dbl[])
            }
          }
        }
      }
      event "test": Value Change {
        n73 = event-data() -> ()  [unwired: 1 in, 6 out]
        n74 = Equal?(x=0.0, y=0.0) -> (x = y?=w253:bool)
        n75 = case shown="True" w253 {
          tunnel: w259 -> [w260 w264]
          tunnel: [w260 w263] -> w258
          tunnel: w256 -> [_ w262]
          frame False {
          }
          frame True {
            n76 = for {
              N: 2 -> [_]
              tunnel: w262 -> [w266]
              shift-right: [w267] -> w263
              shift-left: w264 -> [w268]
              n77 = call "Joystick and Camera SHIH VPC- external Connection.vi"("Motion in"=w268, "XYZTheta"=w266, "Inital GO"=TRUE) -> ("Motion out"=w267:refnum<class "Motion.lvclass">)  [unwired: 4 in, 3 out]
            }
          }
        }
      }
    }
    n78 = feedback-in #1(w28) -> ()
    n79 = feedback-in #2(w26) -> ()
    n80 = feedback-in #3(w25) -> ()
    n81 = feedback-in #4(w13) -> ()
    n82 = feedback-in #5(w29) -> ()
  }
  n83 = call-dynamic "Disconnect.vi"("Controller in"=w8) -> ()  [unwired: 9 in, 1 out]
